vi "CPP-5168PuffAndPressureAnalysis.vi"() -> ()   [LabVIEW 2011]
uses:
  Globals/Plug_in_data_global.vi
  Globals/Meas_global.vi
panel:
  out "Compensated Equi Spaced":dbl[][](array[numeric])
  out "ChannelNames":string[](array[string])
  out "Plug in values":string[](array[string])
  out "Plug in titles":string[](array[string])
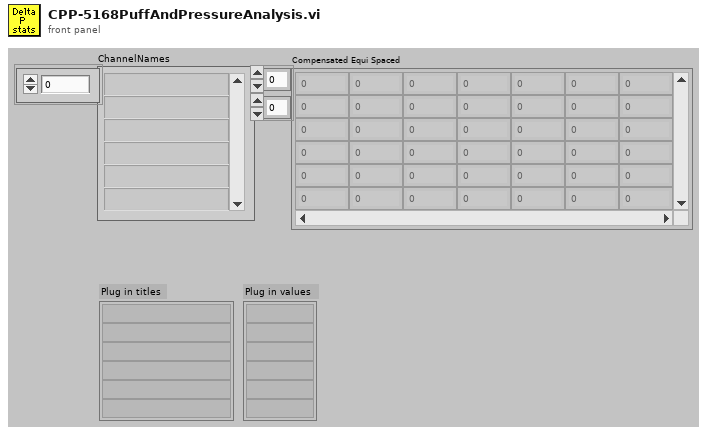
[diagram p1: front panel]
types:
  T1 = typedef "Analysis_info_cluster.ctl" = cluster{"Colour":u32, "Inst type":T2, "Inst name":string, "Symbol":string, "Code name":string, "Extra Info":string, "Inst Array":T3, "Index":i32, "Voltage Index":i32, "Extra Titles":string[], "Extra Values":string[]}
  T2 = typedef "Inst_type.ctl" = enum16{"Propeller anemometer", "Raw voltage", "Pressure Transducer", "Pitot-static tube", "Preston tube", "Hot wire", "Cross wire 1", "Cross wire 2", "Generic Linear", "Generic Polynomial", "Generic BackPoly", "Fast FID", "Thermocouple", "Cold wire", "Pulsed Wire", "LDA Vel", "LDA Tran time", "LDA Arr time"}
  T3 = typedef "Instrument_Array.ctl" = enum16{"PWA", "LDA", "Analogue"}
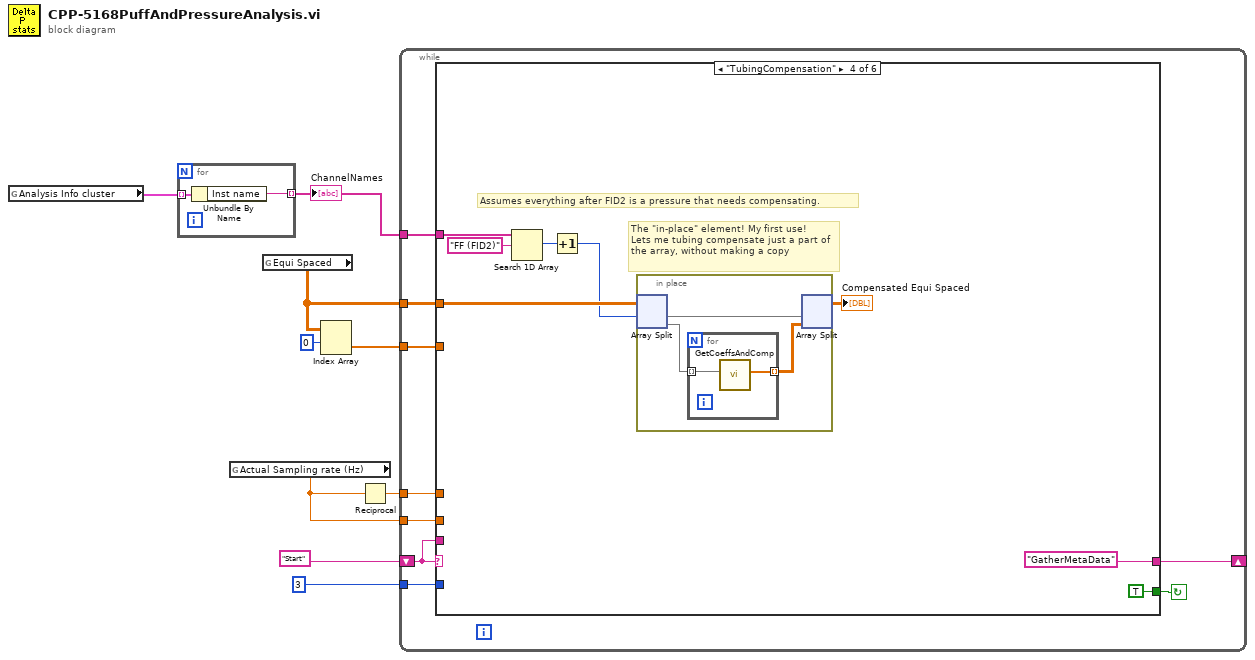
[diagram p0: block diagram]
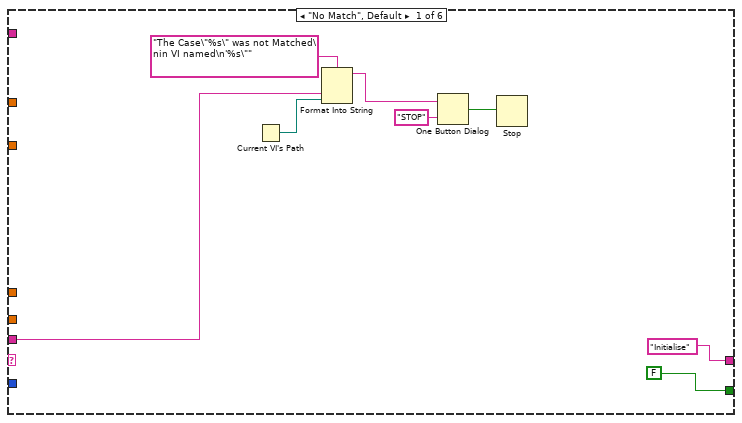
[diagram p2: hidden frame]
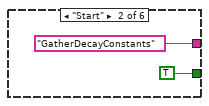
[diagram p3: hidden frame]
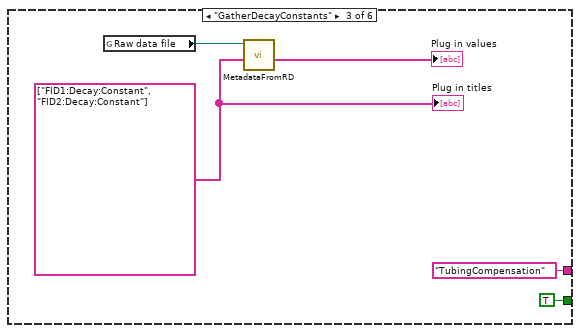
[diagram p4: hidden frame]
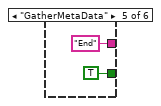
[diagram p5: hidden frame]
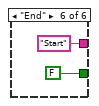
[diagram p6: hidden frame]
diagram:
  n1 = global read "Meas_global.vi" "Analysis Info cluster"() -> (w2:T1[])
  n2 = for {
    tunnel: w2 -> [w11] mode=indexing
    tunnel: [w10] -> w1 mode=indexing
    n3 = Unbundle By Name(w11) -> ("Inst name"=w10:string)
  }
  "ChannelNames" <- w1
  n4 = global read "Meas_global.vi" "Actual Sampling rate (Hz)"() -> (w8:dbl)
  n5 = global read "Plug_in_data_global.vi" "Equi Spaced"() -> (w4:dbl[][])
  n6 = Index Array(array=w4, index (row)=0) -> (element=w3:dbl[])  [unwired: 1 in]
  n7 = Reciprocal(x=w8) -> (1/x=w7:dbl)
  n8 = while {
    shift-left: "Start" -> [w18]
    shift-right: [w19] -> _
    tunnel: w8 -> [w17]
    tunnel: w7 -> [w16]
    tunnel: 3 ("MedianFilter(points)") -> [w15]
    tunnel: w4 -> [w14]
    tunnel: w3 -> [w13]
    tunnel: w1 -> [w12]
    stop <- w20 continue-if-true
    n9 = case shown="\"TubingCompensation\"" w18 {
      tunnel: [FALSE TRUE ("Processing last block?") TRUE ("Processing last block?") TRUE ("Processing last block?") TRUE ("Processing last block?") FALSE ("Processing last block?")] -> w20
      tunnel: ["Initialise" "GatherDecayConstants" "TubingCompensation" ("f") "GatherMetaData" ("f") "End" ("f") "Start" ("f")] -> w19
      tunnel: w18 -> [w23 _ _ _ _ _]
      tunnel: w17 -> [_ _ _ _ _ _]
      tunnel: w16 -> [_ _ _ _ _ _]
      tunnel: w15 -> [_ _ _ _ _ _]
      tunnel: w14 -> [_ _ _ w40 _ _]
      tunnel: w13 -> [_ _ _ _ _ _]
      tunnel: w12 -> [_ _ _ w42 _ _]
      frame "No Match", Default {
        n10 = Current VI's Path() -> (path=w22:path)
        n11 = Format Into String(format string="The Case\"%s\" was not Matched\nin VI named\n'%s\"" ("Format String"), w23, w22) -> (resulting string=w26:string)  [unwired: 2 in, 1 out]
        n12 = One Button Dialog(message=w26, button name ("OK")="STOP") -> (true=w24:bool)
        n13 = Stop(stop? (T)=w24) -> ()
      }
      frame "Start" {
      }
      frame "GatherDecayConstants" {
        w33 = string[] ["FID1:Decay:Constant", "FID2:Decay:Constant"] ("Plug in titles")
        n14 = global read "Meas_global.vi" "Raw data file"() -> (w34:path)
        n15 = call "MetadataFromRD.vi"("ChannelNames"=w33, "Raw data file"=w34) -> ("ValueStrings"=→"Plug in values":string[])  [unwired: 8 in, 1 out]
        "Plug in titles" <- w33
      }
      frame "TubingCompensation" {
        # "The \"in-place\" element! My first use!\nLets me tubing compensate just a part of the array, without making a copy"
        # "Assumes everything after FID2 is a pressure that needs compensating."
        n16 = Search 1D Array(1D array=w42, element="FF (FID2)") -> (index of element=w38:i32)  [unwired: 1 in]
        n17 = Increment(x=w38) -> (x+1=w37:i32)
        n18 = in-place {
          n19 = in-place-split #1(w40, w37) -> (w46:dbl[][], w45:dbl[][])
          n20 = for {
            tunnel: w45 -> [w48] mode=indexing
            tunnel: [w47] -> w44 mode=indexing
            n21 = call "GetCoeffsAndComp.vi"("mutedData"=w48) -> ("boostedData"=w47:dbl[])  [unwired: 10 in]
          }
          n22 = in-place-split #1(w46, w44) -> (→"Compensated Equi Spaced":dbl[][])  [unwired: 1 out]
        }
      }
      frame "GatherMetaData" {
      }
      frame "End" {
      }
    }
  }
